vi "Write Color.vi"(8 "error in (no error)":errorcluster, 10 "Color":u32, 11 "Cluster.lvclass in":refnum<class "Cluster.lvclass">) -> (0 "error out":errorcluster, 3 "Cluster.lvclass out":refnum<class "Cluster.lvclass">)   [LabVIEW 2015, in "Cluster.lvclass"]
uses:
  Cluster.lvclass
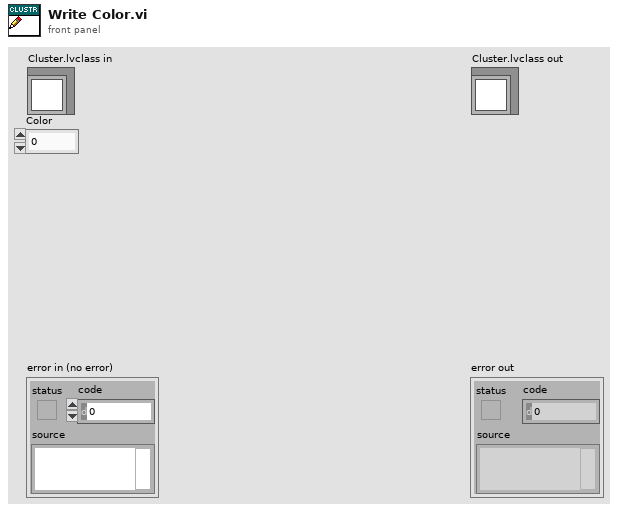
[diagram p1: front panel]
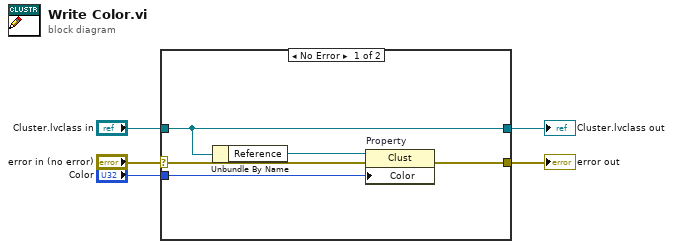
[diagram p0: block diagram]
diagram:
  n1 = case shown="No Error" "error in (no error)" {
    selector: "error in (no error)" -> [w6 w12]
    tunnel: [w10 w12] -> w4
    tunnel: [w8 w11] -> w2
    tunnel: "Cluster.lvclass in" -> [w8 w11]
    tunnel: "Color" -> [w9 _]
    frame No Error {
      n2 = Unbundle By Name(w8) -> ("Reference"=w7:refnum<vi>)
      n3 = property on="Property" class="Clust"(reference=w7, error in=w6, "Color"=w9) -> (error out=w10:errorcluster)  [unwired: 1 out]
    }
    frame Error {
    }
  }
  "error out" <- w4
  "Cluster.lvclass out" <- w2
